vi "Easy2Acquire.IDevice.vi"(0 "IDeviceIn":refnum<k7>, 11 "error in":errorcluster) -> (4 "IDeviceOut":refnum<k7>, 8 "Analog.Select":T1, 10 "GetComponentCount":i32, 13 "Motion.Select":T1=[{"Component"="line.human.pelvis;type.input.motion.rot;device.noraxon.imu.3;", "Collect"=TRUE}, {"Component"="line.human.pelvis.magnetometer.enable;type.command;device.noraxon.imu.3;", "Collect"=FALSE}, {"Component"="line.human.pelvis.magnetometer.disable;type.command;device.noraxon.imu.3;", "Collect"=FALSE}, {"Component"="line.human.pelvis;type.input.motion.accel;device.noraxon.imu.3;", "Collect"=FALSE}, {"Component"="line.magnetometer.reset;device.noraxon.imu.3;type.command;", "Collect"=FALSE}, {"Component"="line.magnetometer.enable;device.noraxon.imu.3;type.command;", "Collect"=FALSE}, {"Component"="line.magnetometer.disable;device.noraxon.imu.3;type.command;", "Collect"=FALSE}], 14 "Digital.Select":T1, 15 "error out":errorcluster)   [LabVIEW 2017]
uses:
  MM-MotionSelect-CTRL.ctl
panel:
  out "IComponent":string[](array[string])
  out "IComponentID":string[](array[string])
  out "IComponentOut":refnum<k7>[](array[refnum])
  out "Components":string[](array[string])
  out "Devices":string[](array[string])
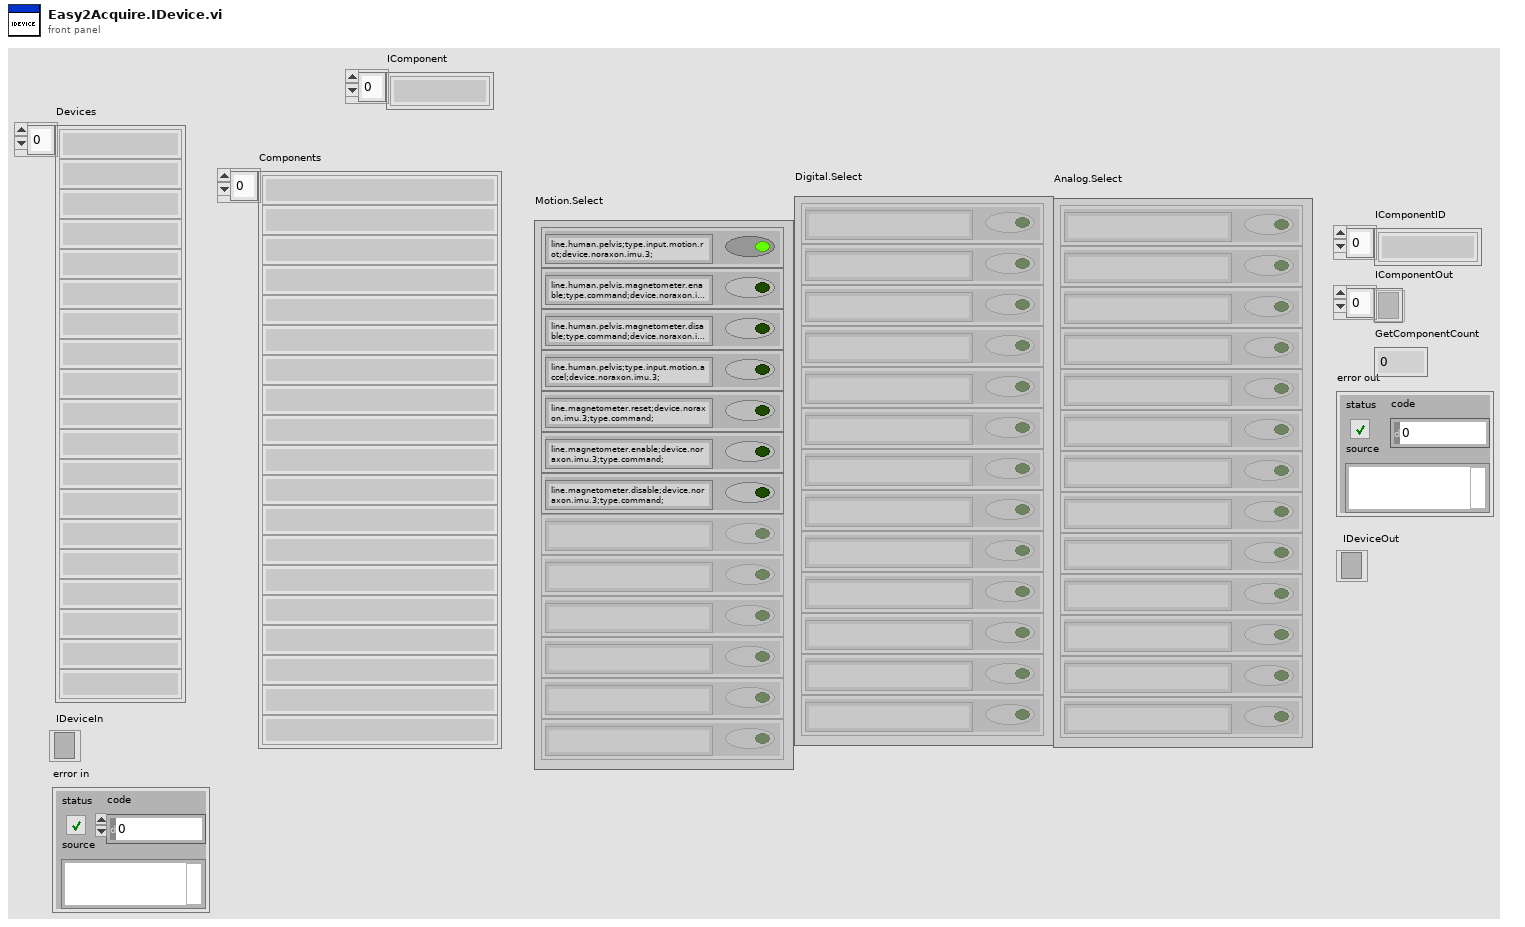
[diagram p1: front panel]
types:
  T1 = typedef "MM-MotionSelect-CTRL.ctl" = cluster{"Component":string, "Collect":bool}[]
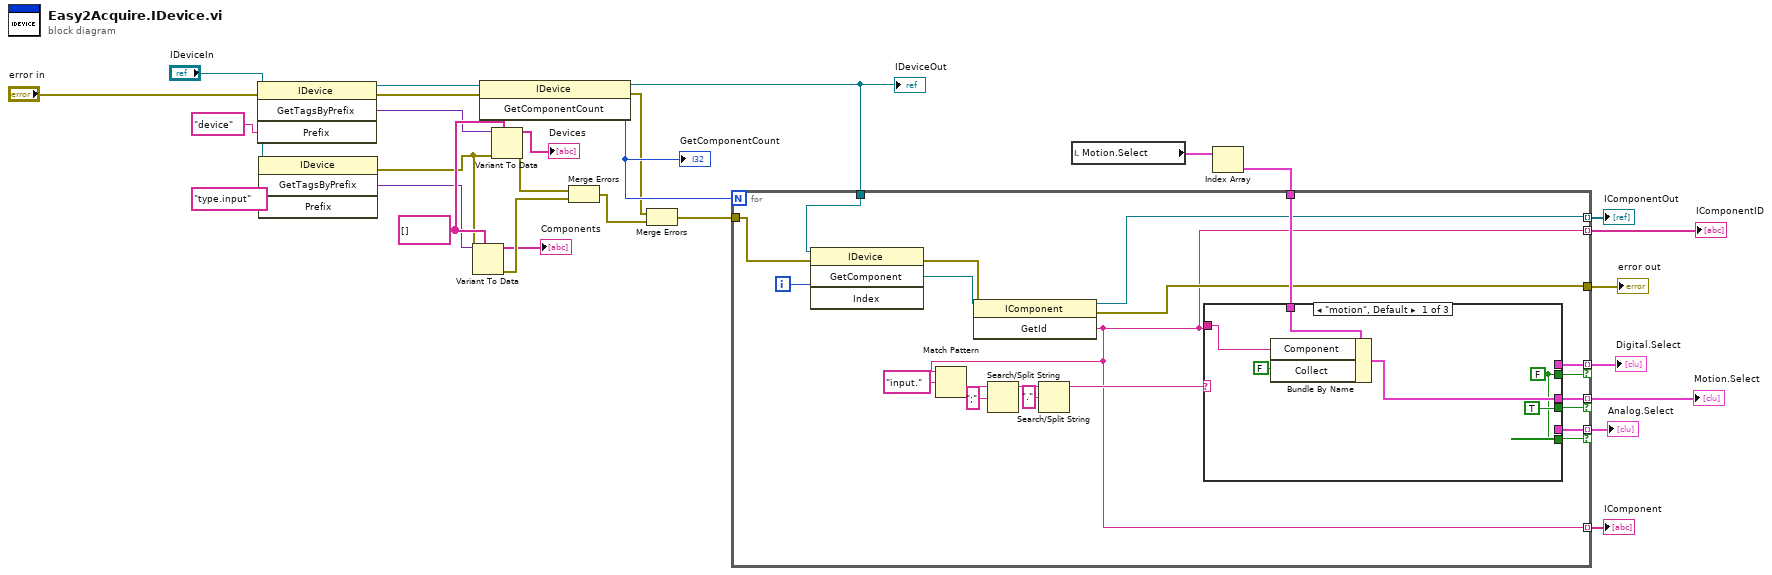
[diagram p0: block diagram]
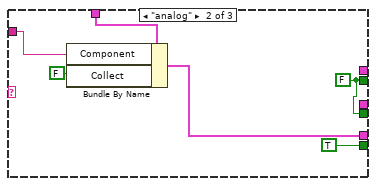
[diagram p2: hidden frame]
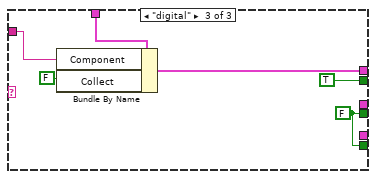
[diagram p3: hidden frame]
diagram:
  w28 = string[] []
  n1 = invoke class="IDevice" method="GetTagsByPrefix"(reference="IDeviceIn", error in="error in", "Prefix"="device") -> (reference out=w15:refnum<k7>, error out=w16:errorcluster, "GetTagsByPrefix"=w19:variant)  [unwired: 1 in, 1 out]
  n2 = invoke class="IDevice" method="GetTagsByPrefix"(reference="IDeviceIn", "Prefix"="type.input") -> (error out=w26:errorcluster, "GetTagsByPrefix"=w23:variant)  [unwired: 2 in, 2 out]
  n3 = Variant To Data(error in=w26, type=w28, Variant=w23) -> (data=→"Components":string[], error out=w25:errorcluster)
  n4 = invoke class="IDevice" method="GetComponentCount"(reference=w15, error in=w16) -> (reference out=w8:refnum<k7>, error out=w10:errorcluster, "GetComponentCount"=w14:i32)  [unwired: 1 in]
  "IDeviceOut" <- w8
  "GetComponentCount" <- w14
  n5 = Variant To Data(error in=w26, type=w28, Variant=w19) -> (data=→"Devices":string[], error out=w27:errorcluster)
  n6 = Merge Errors(w27, w25) -> (w11:errorcluster)
  n7 = Merge Errors(w10, w11) -> (w9:errorcluster)
  n8 = local read "Motion.Select"() -> (w2:T1)
  n9 = Index Array(array=w2) -> (element=w1:cluster{"Component":string, "Collect":bool})  [unwired: 1 in]
  n10 = for {
    N: w14 -> [_]
    tunnel: w1 -> [w40]
    tunnel: [w39] -> w13 mode=indexing if=w38
    tunnel: [w37] -> w4 mode=indexing if=w36
    tunnel: [w35] -> w12 mode=indexing if=w34
    tunnel: w9 -> [w33]
    tunnel: w8 -> [w32]
    tunnel: [w31] -> w7 mode=indexing
    tunnel: [w29] -> w6 mode=indexing
    tunnel: [w30] -> w5
    tunnel: [w29] -> w3 mode=indexing
    i -> [w47]
    n11 = invoke class="IDevice" method="GetComponent"(reference=w32, error in=w33, "Index"=w47) -> (error out=w48:errorcluster, "GetComponent"=w49:refnum<k7>)  [unwired: 1 in, 2 out]
    n12 = invoke class="IComponent" method="GetId"(reference=w49, error in=w48) -> (reference out=w31:refnum<k7>, error out=w30:errorcluster, "GetId"=w29:string)  [unwired: 1 in]
    n13 = Match Pattern(string=w29, regular expression="input.") -> (after substring=w45:string)  [unwired: 1 in, 3 out]
    n14 = Search/Split String(string=w45, search string/char (-)=";" ("regular expression")) -> (substring before match=w43:string)  [unwired: 1 in, 2 out]
    n15 = Search/Split String(string=w43, search string/char (-)=".") -> (substring before match=w41:string)  [unwired: 1 in, 2 out]
    n16 = case shown="\"motion\", Default" w41 {
      tunnel: w29 -> [w54 w60 w66]
      tunnel: w40 -> [w52 w59 w67]
      tunnel: [_ _ w64] -> w39
      tunnel: [w50 w57 TRUE ("Collect")] -> w38
      tunnel: [w53 _ _] -> w37
      tunnel: [TRUE w57 w62] -> w36
      tunnel: [_ w58 _] -> w35
      tunnel: [w50 TRUE w62] -> w34
      frame "motion", Default {
        w50 = FALSE ("Collect")
        n17 = Bundle By Name(cluster=w52, "Component"=w54, "Collect"=FALSE) -> (w53:cluster{"Component":string, "Collect":bool})
      }
      frame "analog" {
        w57 = FALSE ("Collect")
        n18 = Bundle By Name(cluster=w59, "Component"=w60, "Collect"=FALSE) -> (w58:cluster{"Component":string, "Collect":bool})
      }
      frame "digital" {
        w62 = FALSE ("Collect")
        n19 = Bundle By Name(cluster=w67, "Component"=w66, "Collect"=FALSE) -> (w64:cluster{"Component":string, "Collect":bool})
      }
    }
  }
  "error out" <- w5
  "Motion.Select" <- w4
  "Digital.Select" <- w13
  "Analog.Select" <- w12
  "IComponentOut" <- w7
  "IComponentID" <- w6
  "IComponent" <- w3
